vi "Read Temperature.vi"(8 "error in (no error)":errorcluster, 11 "VISA resource name":refnum<visa-resource-name>) -> (0 "error out":errorcluster, 2 "Control Temperature":dbl format="%#.1g", 3 "VISA resource name out":refnum<visa-resource-name>)   [LabVIEW 2010, in "Temptronic TP04300.lvlib"]
doc: "This VI reads the main control (air in air mode or DUT in the DUT mode)temperature in Celsius."
uses:
  Temptronic TP04300.lvlib
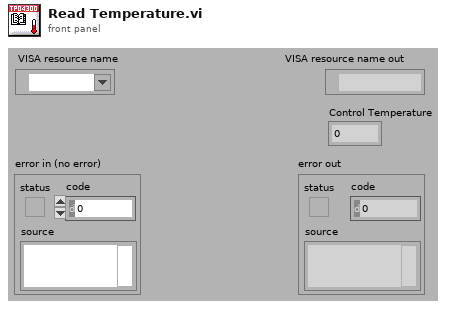
[diagram p1: front panel]
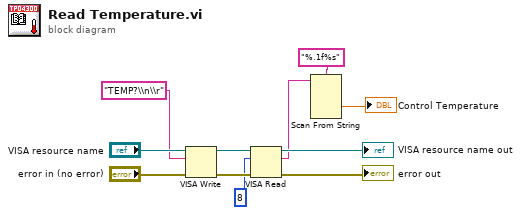
[diagram p0: block diagram]
diagram:
  n1 = VISA Write(VISA resource name="VISA resource name", write buffer="TEMP?\\n\\r" ("multi-line string"), error in (no error)="error in (no error)") -> (VISA resource name out=w7:refnum<visa-resource-name>, error out=w9:errorcluster)  [unwired: 1 out]
  n2 = VISA Read(VISA resource name=w7, byte count=u32 8, error in (no error)=w9) -> (VISA resource name out=→"VISA resource name out":refnum<visa-resource-name>, read buffer=w3:string, error out=→"error out":errorcluster)  [unwired: 1 out]
  n3 = Scan From String(format string="%.1f%s" ("multi-line string"), input string=w3) -> (output 1=→"Control Temperature":dbl)  [unwired: 5 in, 3 out]
